vi "Read Engine Period.vi"(8 "error in (no error)":errorcluster, 11 "Simulated VeriStand Engine in":refnum<class "Simulated VeriStand Engine.lvclass">) -> (0 "error out":errorcluster, 2 "Engine Period":u32 format="%d us", 3 "Simulated VeriStand Engine out":refnum<class "Simulated VeriStand Engine.lvclass">)   [LabVIEW 2016, in "Simulated VeriStand Engine.lvclass"]
uses:
  Simulated VeriStand Engine.lvclass
  Simulated VeriStand Engine.lvclass/Simulated VeriStand Engine.ctl
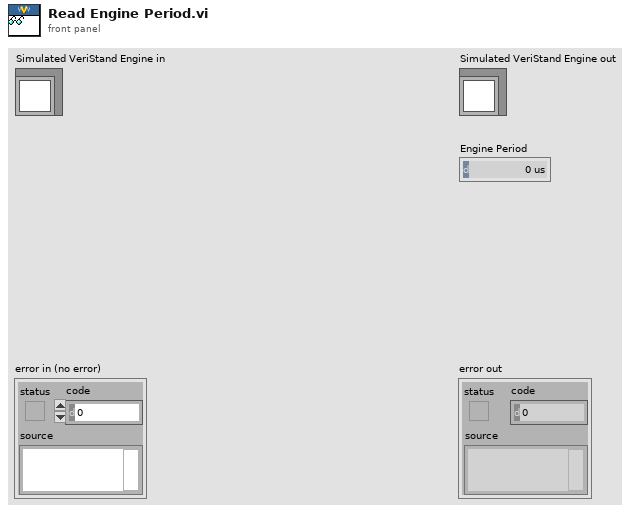
[diagram p1: front panel]
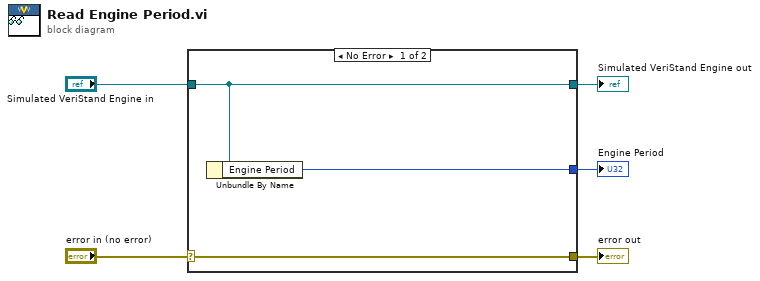
[diagram p0: block diagram]
diagram:
  n1 = case shown="No Error" "error in (no error)" {
    selector: "error in (no error)" -> [w8 w9]
    tunnel: [w8 w9] -> w4
    tunnel: [w7 w10] -> w2
    tunnel: "Simulated VeriStand Engine in" -> [w7 w10]
    tunnel: [w6 _] -> w1
    frame No Error {
      n2 = Unbundle By Name(w7) -> ("Engine Period"=w6:u32)
    }
    frame Error {
    }
  }
  "error out" <- w4
  "Simulated VeriStand Engine out" <- w2
  "Engine Period" <- w1
